vi "Get_Device_ID.vi"(8 "错误输入":errorcluster) -> (0 "错误输出":errorcluster, 3 "Device_ID":string)   [LabVIEW 2018]
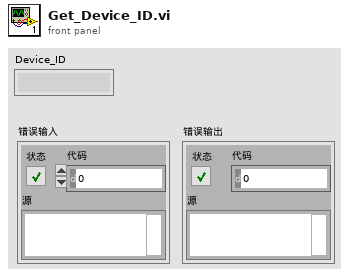
[diagram p1: front panel]
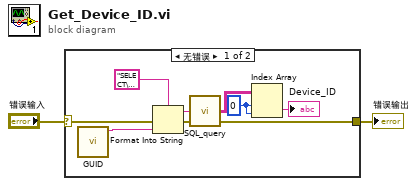
[diagram p0: block diagram]
diagram:
  n1 = case shown="无错误" "错误输入" {
    selector: "错误输入" -> [w8 w12]
    tunnel: [w6 w12] -> w1
    frame No Error {
      w10 = 0 ("索引 (行)")
      n2 = call "GUID.vi"() -> ("trimmed string"=w4:string)  [unwired: 11 in]
      n3 = Format Into String(format string="SELECT\ndbo.Device.DEVICE_ID\n\nFROM\ndbo.Device\nWHERE\ndbo.Device.DEVICE_PC_ID = '%s'\n", error in=w8, w4) -> (resulting string=w11:string, error out=w7:errorcluster)  [unwired: 1 in]
      n4 = call "SQL_query.vi"("error in (no error)"=w7, "SQL query"=w11) -> ("error out"=w6:errorcluster, "data"=w5:string[][])  [unwired: 1 in, 1 out]
      n5 = Index Array(array=w5, index (row)=w10, index (col)=w10) -> (element=→"Device_ID":string)
    }
    frame Error {
    }
  }
  "错误输出" <- w1
